vi "CompVisionUtil_CalculateDistanceToTarget.vi"(8 "targetPitch_Radians":dbl, 9 "cameraPitch_Radians":dbl, 10 "targetHeight_Meters":dbl, 11 "cameraHeight_Meters":dbl) -> (3 "DistanceToTarget_Meters":dbl)   [LabVIEW 2019, in "Trajectory_Library.lvlib"]
doc: "Algorithm from https://docs.limelightvision.io/en/latest/cs_estimating_distance.html Estimates range to a target using the target's elevation. This method can produce more stable results than SolvePNP when well tuned, if the full 6d robot pose is not required. Note that this method requires the camera to have 0 roll (not be skewed clockwise or CCW relative to the floor), and for there to exist a height differential between goal and camera. The larger this differential, the more accurate the distance estimate will be.\n \nUnits can be converted using the conversion functions.\n \nInputs:\n - CameraHeight_Meters -- The physical height of the camera off the floor \n in meters.\n - TargetHeightMeters -- The physical height of the target off the floor in meters. \n This should be the height of whatever is being targeted (i.e. if the \n targeting region is set to top, this should be the height of the top \n of the target).\n - CameraPitch_Radians -- The pitch of the camera from the horizontal plane \n in radians.\n Positive values up.\n - TargetPitchRadian -- The pitch of the target in the camera's lens in radians. \n Positive values up.\n\nOutputs\n - DistanceToTarget_Meters -- The estimated distance to the target in meters."
uses:
  Trajectory_Library.lvlib
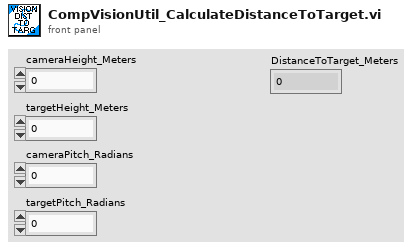
[diagram p1: front panel]
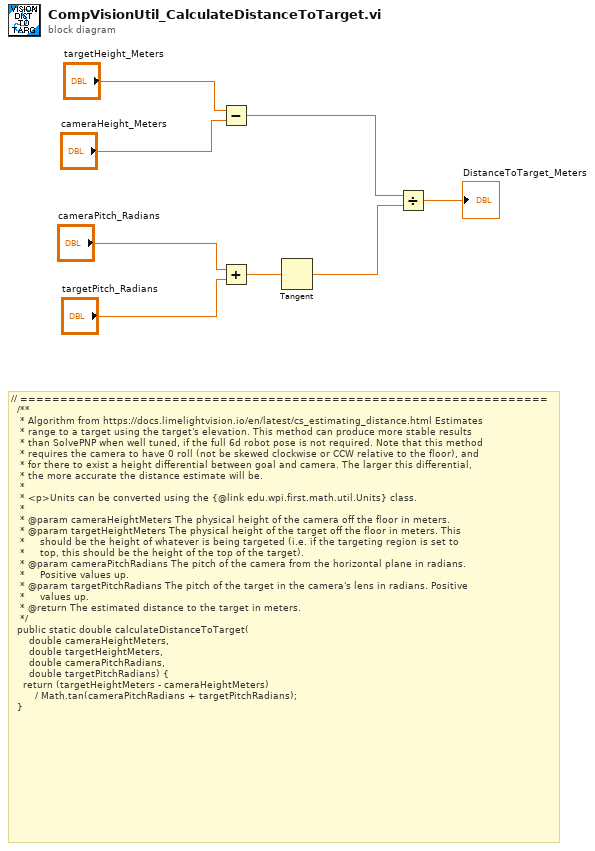
[diagram p0: block diagram]
diagram:
  # "// ==================================================================\n  /**\n   * Algorithm from https://docs.limelightvision.io/en/latest/cs_estimating_distance.html Estimates\n   * range to a target using the target's elevation. This method can produce more stable results\n   * than SolvePNP when well tuned, if the full 6d robot pose is not required. Note that this method\n   * requires the camera to have 0 roll (not be skewed clockwise or CCW relative to the floor), and\n   * for there to exist a height differential between goal and camera. The larger this differential,\n   * the more accurate the distance estimate will be.\n   *\n   * <p>Units can be converted using the {@link edu.wpi.first.math.util.Units} class.\n   *\n   * @param cameraHeightMeters The physical height of the camera off the floor in meters.\n   * @param targetHeightMeters The physical height of the target off the floor in meters. This\n   *     should be the height of whatever is being targeted (i.e. if the targeting region is set to\n   *     top, this should be the height of the top of the target).\n   * @param cameraPitchRadians The pitch of the camera from the horizontal plane in radians.\n   *     Positive values up.\n   * @param targetPitchRadians The pitch of the target in the camera's lens in radians. Positive\n   *     values up.\n   * @return The estimated distance to the target in meters.\n   */\n  public static double calculateDistanceToTarget(\n      double cameraHeightMeters,\n      double targetHeightMeters,\n      double cameraPitchRadians,\n      double targetPitchRadians) {\n    return (targetHeightMeters - cameraHeightMeters)\n        / Math.tan(cameraPitchRadians + targetPitchRadians);\n  }"
  n1 = Subtract(x="targetHeight_Meters", y="cameraHeight_Meters") -> (x-y=w7:dbl)
  n2 = Add(x="cameraPitch_Radians", y="targetPitch_Radians") -> (x+y=w8:dbl)
  n3 = Tangent(1:w8) -> (0:w6:dbl)
  n4 = Divide(x=w7, y=w6) -> (x/y=→"DistanceToTarget_Meters":dbl)
